vi "Wait for Acquisition Complete.vi"(7 "Maximum Time (10000 ms)":u32=10000, 8 "error in (no error)":errorcluster, 9 "Number of Points (100)":u32=100, 11 "VISA resource name":refnum<visa-resource-name>) -> (0 "error out":errorcluster, 3 "VISA resource name out":refnum<visa-resource-name>)   [LabVIEW 2023, in "Stanford Research 830.lvlib"]
doc: "Waits for the number of pointed desired to complete. This VI should be called after Start VI and before Fetch Buffer VI.\n\n<B>Note:</B> \n\nUse this VI only with other low-level VIs. The high-level VIs automatically incorporate this functionality. This VI does not check the instrument status."
uses:
  Stanford Research 830.lvlib
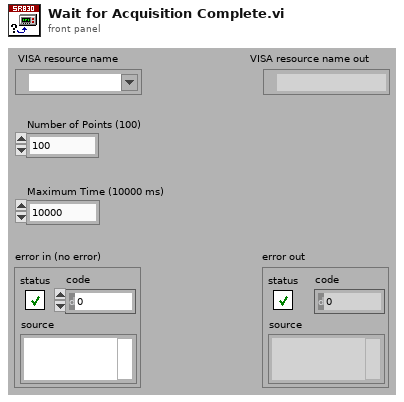
[diagram p1: front panel]
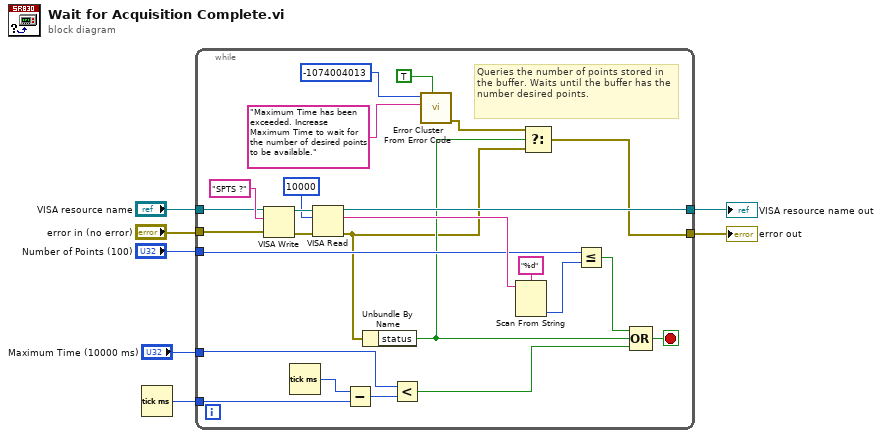
[diagram p0: block diagram]
diagram:
  n1 = Tick Count (ms)() -> (millisecond timer value=w4:u32)
  n2 = while {
    tunnel: [w26] -> w2
    tunnel: [w8] -> w1
    tunnel: "error in (no error)" -> [w24]
    tunnel: "VISA resource name" -> [w23]
    tunnel: "Number of Points (100)" -> [w22]
    tunnel: w4 -> [w19]
    tunnel: "Maximum Time (10000 ms)" -> [w18]
    stop <- w15 stop-if-true
    # "Queries the number of points stored in the buffer. Waits until the buffer has the number desired points."
    n3 = VISA Write(VISA resource name=w23, write buffer="SPTS ?", error in (no error)=w24) -> (VISA resource name out=w32:refnum<visa-resource-name>, error out=w31:errorcluster)  [unwired: 1 out]
    n4 = Tick Count (ms)() -> (millisecond timer value=w20:u32)
    n5 = VISA Read(VISA resource name=w32, byte count=u32 10000, error in (no error)=w31) -> (VISA resource name out=w26:refnum<visa-resource-name>, read buffer=w28:string, error out=w13:errorcluster)  [unwired: 1 out]
    n6 = Subtract(x=w20, y=w19) -> (x-y=w21:u32)
    n7 = Unbundle By Name(w13) -> ("status"=w14:bool)
    n8 = Less?(x=w18, y=w21) -> (x < y?=w16:bool)
    n9 = call <vilib>:"Error Cluster From Error Code.vi"("show call chain? (False)"=TRUE, "error message (\"\")"="Maximum Time has been exceeded. Increase Maximum Time to wait for the number of desired points to be available." ("error message (\"\")"), "error code (0)"=-1074004013) -> ("error out"=w9:errorcluster)  [unwired: 6 in]
    n10 = Scan From String(format string="%d", input string=w28) -> (output 1=w25:i32)  [unwired: 3 in, 3 out]
    n11 = Select(t=w9, s=w14, f=w13) -> (s? t:f=w8:errorcluster)
    n12 = Less Or Equal?(x=w22, y=w25) -> (x <= y?=w17:bool)
    n13 = Compound Arithmetic op=OR(w17, w14, w16) -> (w15:bool)
  }
  "error out" <- w1
  "VISA resource name out" <- w2
